vi "Execute.vi"(1 "Numeric":dbl, 4 "Position":i32, 6 "Assembly Type":string, 8 "error in (no error)":errorcluster, 9 "Workspace":T1, 10 "Cluster":T2={"I-O.lvclass"=refnum, "Gantry"=refnum, "Dispenser"="COM1"}, 11 "Pick and Place in":refnum<class "Pick and Place.lvclass">) -> (0 "error out":errorcluster, 2 "Control Out":T2={"I-O.lvclass"=refnum, "Gantry"=refnum, "Dispenser"="COM1"}, 3 "Pick and Place out":refnum<class "Pick and Place.lvclass">)   [LabVIEW 2021, in "Pick and Place.lvclass"]
uses:
  Pick and Place.lvclass
  Controller/Controllers.ctl
  Controller/I-O/I-O.lvclass
  C:/Program Files (x86)/Aerotech/A3200/LabVIEW/2010/Bin/Aerotech.A3200.dll
  Program Files (x86)/Aerotech/A3200/LabVIEW/2010/Bin/Aerotech.A3200.dll
  Workspace/Workspace.ctl
  Pick and Place.lvclass/Pick and Place.ctl
  Pick and Place Type.ctl
  Drivers/Aerotech A3200/Parameters/GetAxisParameterDouble.vi
  Controller/Motion/Motion.lvclass
  Controller/Motion/A3200/A3200.lvclass
  Drivers/Aerotech A3200/Aerotech.lvlib
  Controller/Controller.lvclass
  Workspace/Fixture.lvclass
panel:
  out "Seconary Pickup time 2":timestamp
  out "Seconary Pickup time 1":timestamp
  out "milliseconds to wait":u32
  out "XYZTheta Out":dbl[](array[numeric])
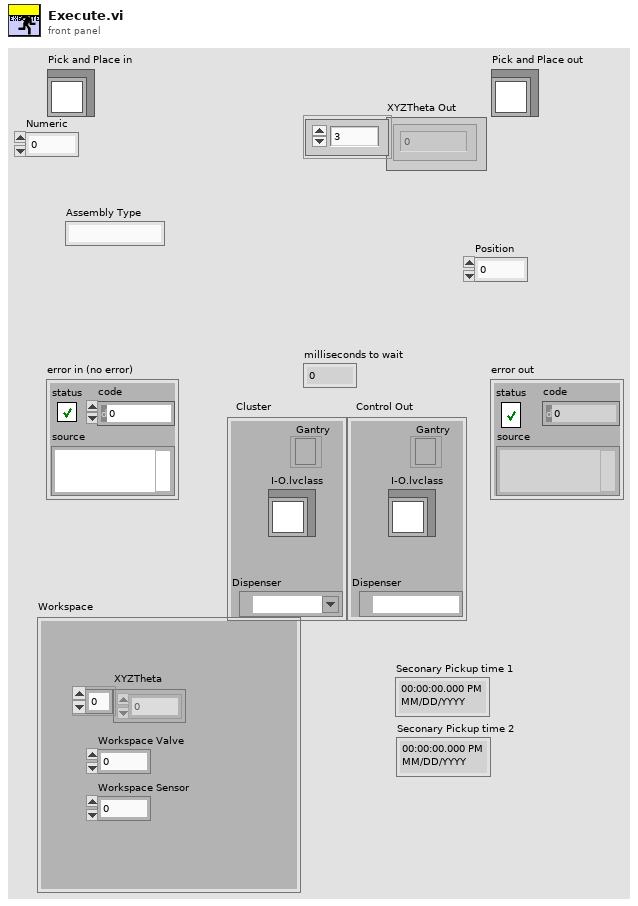
[diagram p1: front panel]
types:
  T1 = typedef "Fixture.lvclass/Workspace.ctl" = cluster{"XYZTheta":dbl[], "Workspace Valve":i32, "Workspace Sensor":i32}
  T2 = typedef "Controller.lvclass/Controllers.ctl" = cluster{"I-O.lvclass":refnum<class "I-O.lvclass">, "Gantry":refnum<k24>, "Dispenser":refnum<visa-resource-name>}
  T3 = typedef "I-O.lvclass/Pin Map.ctl" = cluster{"Region Valves":i32[], "Extra Valves":dbl[][][], "Tool Primary Valve":i32, "Tool Secondary Valve":i32, "Region Sensors":i32[], "Extra Sensors":dbl[][][], "Tool Primary Sensor":dbl, "Tool Secondary Sensor":dbl, "Compression Sensor":dbl, "5V":i32, "Dispenser Sensor":dbl}
  T4 = typedef "Pick and Place.lvclass/Pick and Place Type.ctl" = enum16{"Primary Pick Up", "Secondary Pick Up", "Put Down All", "Pick Up All", "Put Down Secondary"}
  T5 = cluster{"Status":bool, "Error Code":i32, "Source":string}
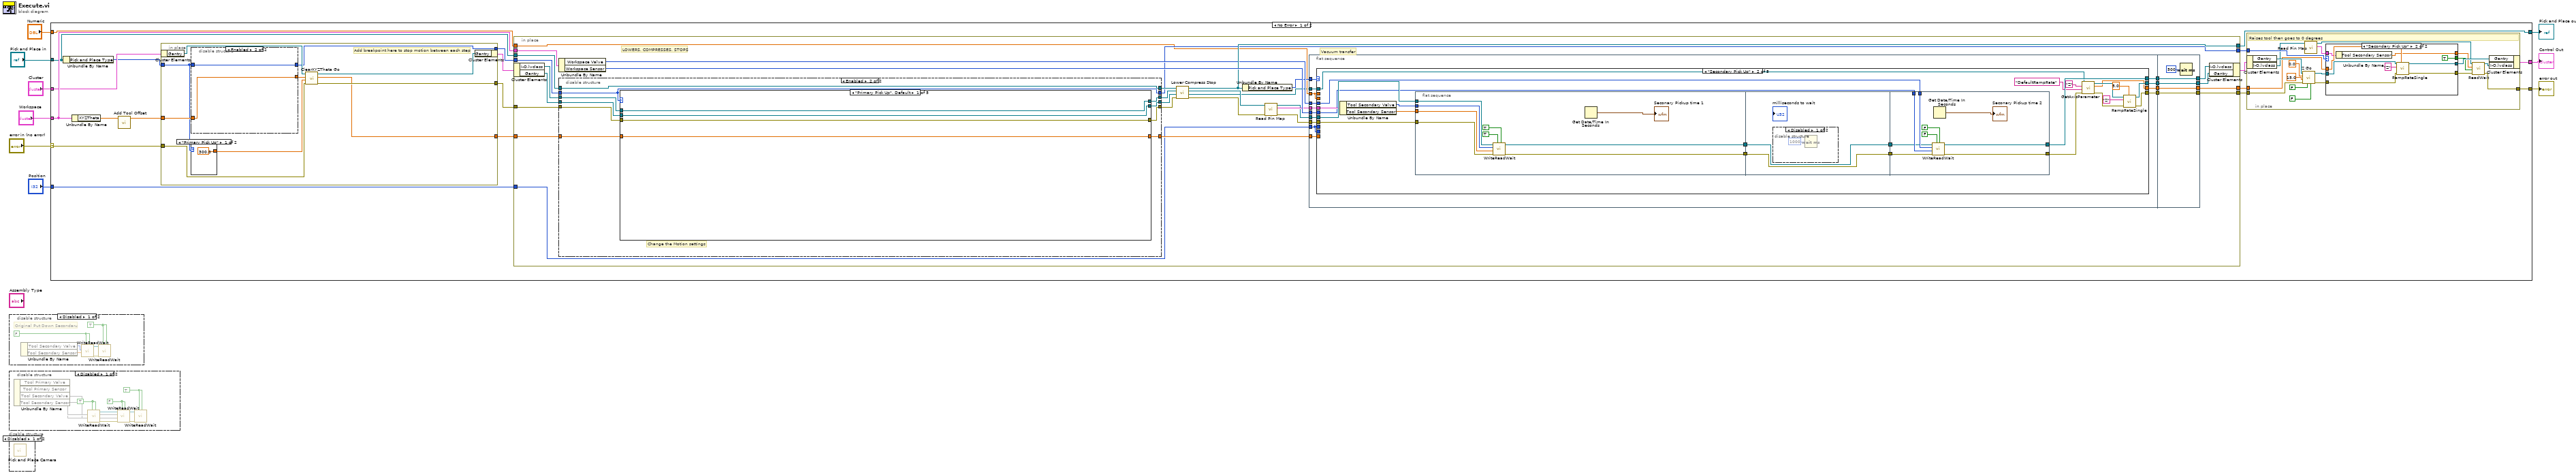
[diagram p0: block diagram]
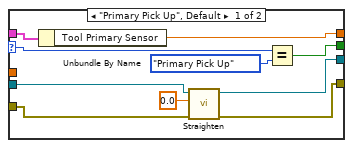
[diagram p5: hidden frame]
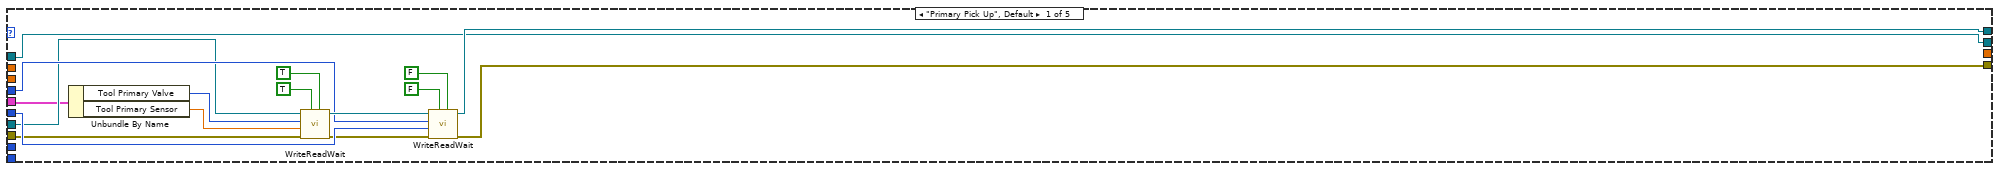
[diagram p6: hidden frame]
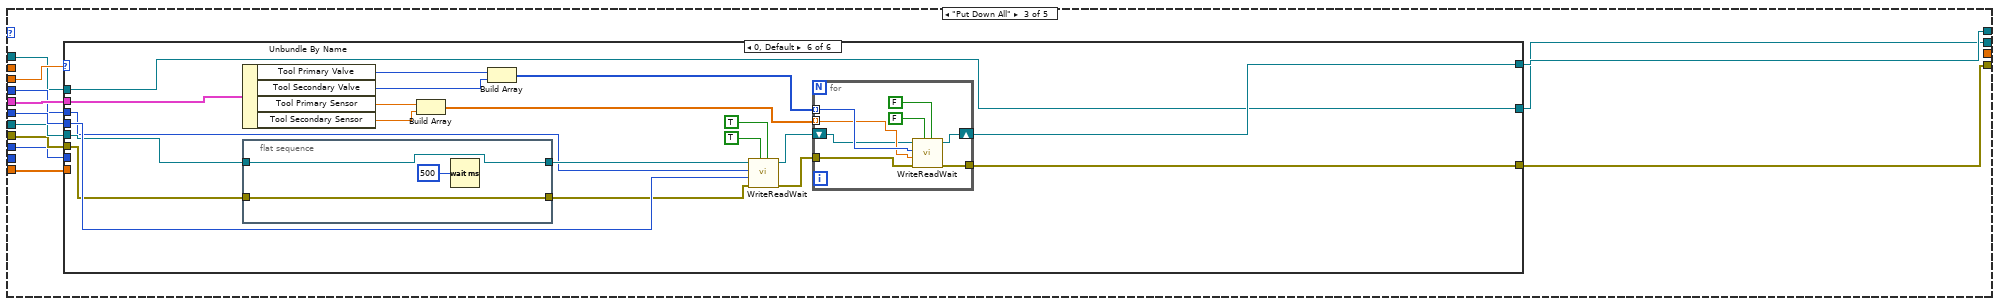
[diagram p8: hidden frame]
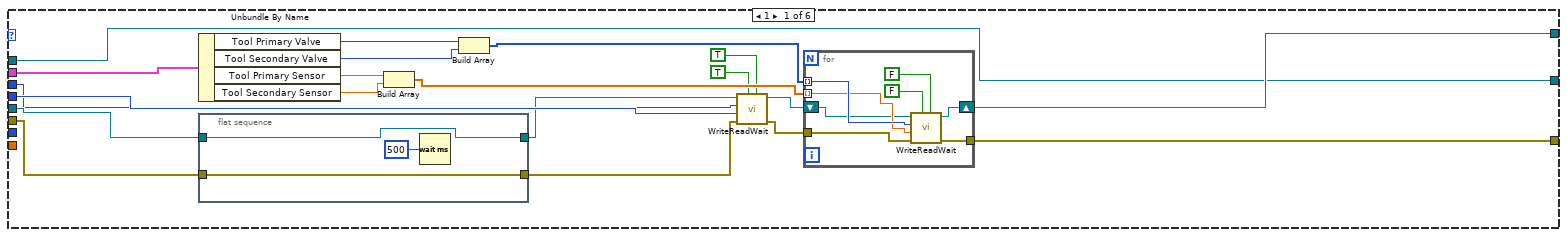
[diagram p9: hidden frame]
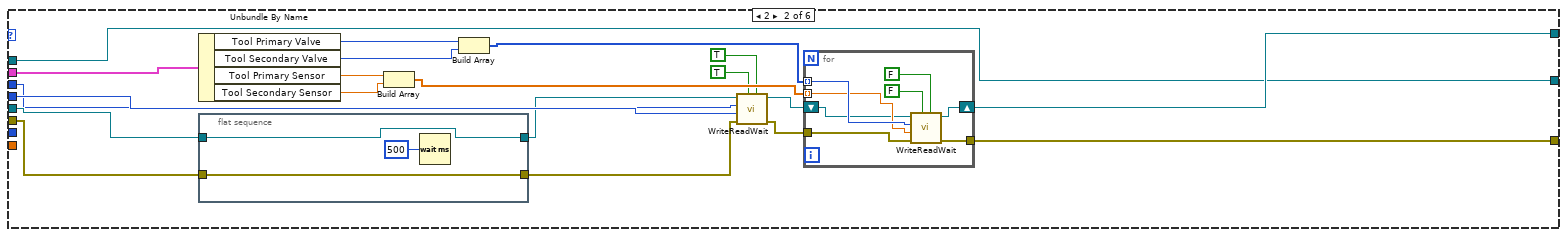
[diagram p10: hidden frame]
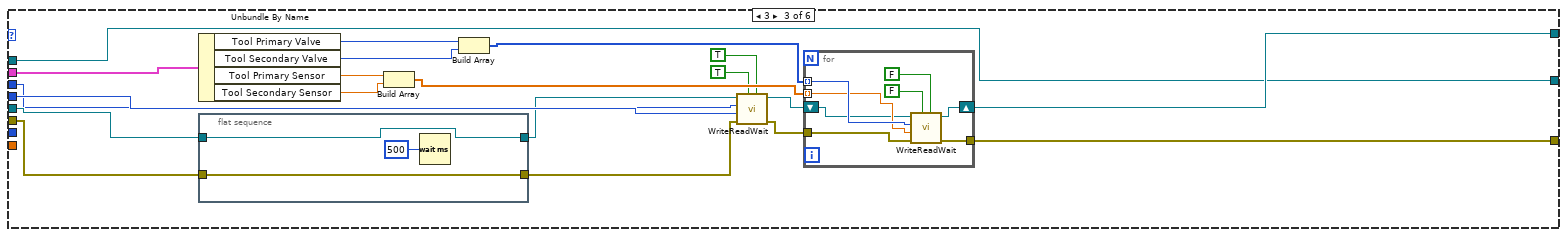
[diagram p11: hidden frame]
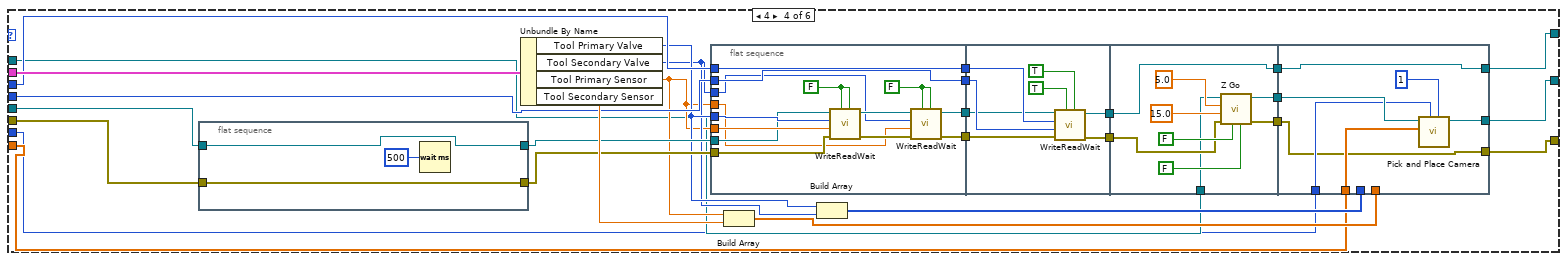
[diagram p12: hidden frame]
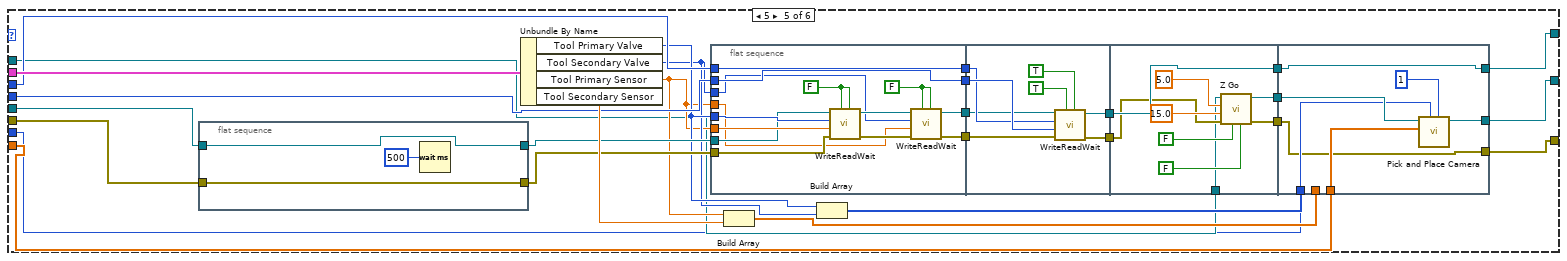
[diagram p13: hidden frame]
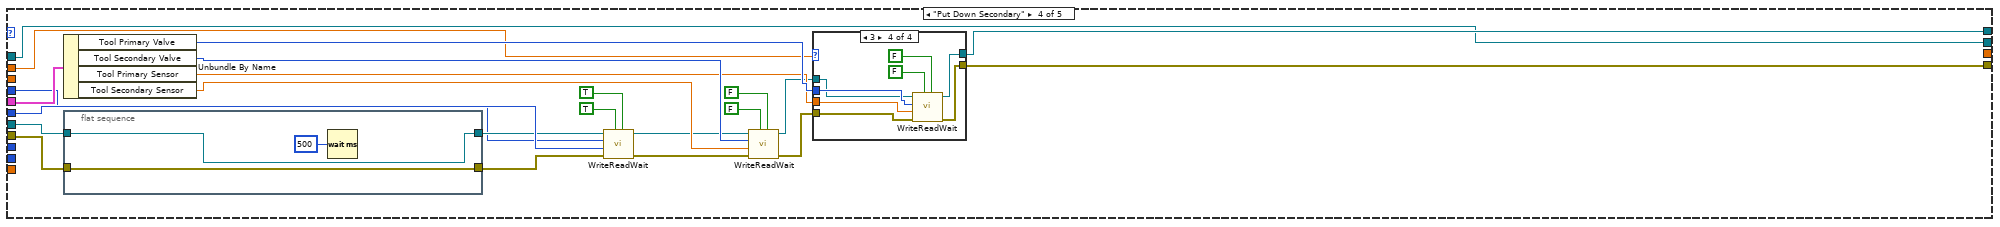
[diagram p14: hidden frame]
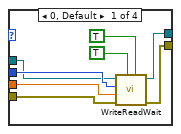
[diagram p15: hidden frame]
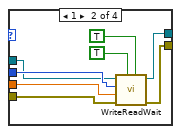
[diagram p16: hidden frame]
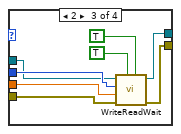
[diagram p17: hidden frame]
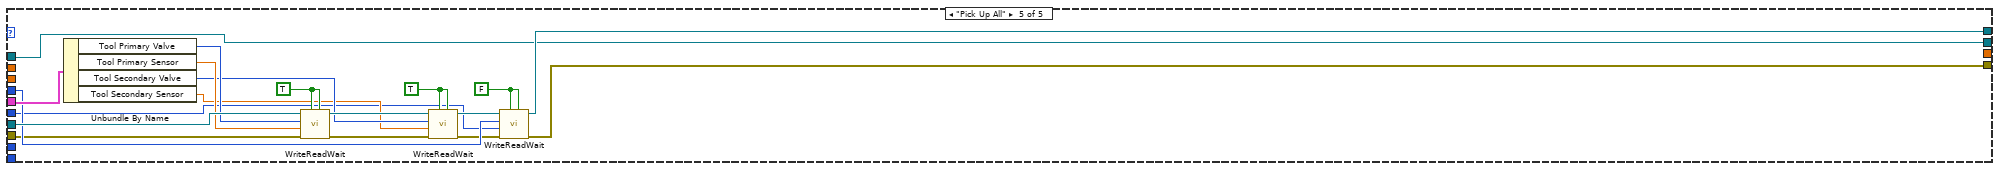
[diagram p18: hidden frame]
diagram:
  n1 = disable-structure shown="Disabled" {
    frame Disabled {
      w14 = TRUE ("Read Value")
      w18 = FALSE ("Write Value")
      # "Original Put Down Secondaru"
      n2 = Unbundle By Name() -> ("Tool Secondary Valve"=w20:i32, "Tool Secondary Sensor"=w19:dbl)  [unwired: 1 in]
      n3 = call "WriteReadWait.vi"("Read Value"=w18, "Write Value"=w18, "Read"=w19, "Write"=w20) -> ("error out"=w11:errorcluster, "I-O out"=w17:refnum<class "I-O.lvclass">, "error in (no error)"=w12:errorcluster, "I-O in"=w21:refnum<class "I-O.lvclass">)  [unwired: 4 in]
      n4 = call "WriteReadWait.vi"("Read Value"=w14, "Write Value"=w14, "error in (no error)"=w11, "I-O in"=w17) -> ("error out"=w10:errorcluster, "I-O out"=w13:refnum<class "I-O.lvclass">, "Read"=w15:i32, "Write"=w16:i32)  [unwired: 4 in]
    }
    frame Enabled {
    }
  }
  n5 = disable-structure shown="Disabled" {
    frame Disabled {
      w27 = TRUE ("Read Value")
      w31 = FALSE ("Write Value")
      w37 = TRUE ("Write Value")
      n6 = Unbundle By Name() -> (w39:T3, "Tool Primary Valve"=w36, "Tool Primary Sensor"=w35, "Tool Secondary Valve"=w33, "Tool Secondary Sensor"=w32)
      n7 = call "WriteReadWait.vi"("Read Value"=w37, "Write Value"=w37, "Read"=w35, "Write"=w36) -> ("error out"=w24:errorcluster, "I-O out"=w34:refnum<class "I-O.lvclass">, "error in (no error)"=w25:errorcluster, "I-O in"=w38:refnum<class "I-O.lvclass">)  [unwired: 4 in]
      n8 = call "WriteReadWait.vi"("Read Value"=w31, "Write Value"=w31, "error in (no error)"=w24, "Read"=w32, "Write"=w33, "I-O in"=w34) -> ("error out"=w23:errorcluster, "I-O out"=w30:refnum<class "I-O.lvclass">)  [unwired: 4 in]
      n9 = call "WriteReadWait.vi"("Read Value"=w27, "Write Value"=w27, "error in (no error)"=w23, "I-O in"=w30) -> ("error out"=w22:errorcluster, "I-O out"=w26:refnum<class "I-O.lvclass">, "Read"=w28:i32, "Write"=w29:i32)  [unwired: 4 in]
    }
    frame Enabled {
    }
  }
  n10 = disable-structure shown="Disabled" {
    frame Disabled {
      n11 = call "Pick and Place Camera.vi"() -> ("Gantry In"=w40:refnum<k24>, "XYZTheta"=w41:dbl[], "Position"=w44:i32, "Tray Number"=w43:i32, "Gantry Out"=w42:refnum<k24>)  [unwired: 6 in]
    }
    frame Enabled {
    }
  }
  n12 = case shown="No Error" "error in (no error)" {
    selector: "error in (no error)" -> [w58 w662]
    tunnel: "Cluster" -> [w62 w663]
    tunnel: "Workspace" -> [w63 _]
    tunnel: [w57 w662] -> w3
    tunnel: [w61 w663] -> w4
    tunnel: "Pick and Place in" -> [w53 w661]
    tunnel: [w60 w661] -> w8
    tunnel: "Numeric" -> [w47 _]
    tunnel: "Position" -> [w46 _]
    frame No Error {
      n13 = Unbundle By Name(w53) -> ("Pick and Place Type"=w52:T4)
      n14 = Unbundle By Name(w63) -> ("XYZTheta"=w49:dbl[])
      n15 = call "Add Tool Offset.vi"("XYZTheta"=w49) -> ("Array"=w59:dbl[])  [unwired: 10 in]
      n16 = in-place "In Place Element Structure" {
        in-place-border: w59 -> [w642]
        in-place-border: w58 -> [w643]
        in-place-border: [w644] -> w55
        in-place-border: w52 -> [w638]
        in-place-border: [w640] -> w51
        in-place-border: [w639] -> w48
        # "Add breakpoint here to stop motion between each step"
        n17 = in-place-cluster #1(w62) -> ("Gantry"=w646:refnum<k24>)
        n18 = disable-structure shown="Enabled" {
          disable-tunnel: w638 -> [w649 w659]
          disable-tunnel: w642 -> [w651 w660]
          disable-tunnel: [w650 w660] -> w641
          disable-tunnel: [w649 w659] -> w640
          frame Disabled {
            n19 = case shown="\"Put Down All\"" w649 {
              tunnel: w651 -> [w652 w655]
              tunnel: [w652 w653] -> w650
              frame "Primary Pick Up", Default {
              }
              frame "Put Down All" {
                n20 = in-place {
                  n21 = in-place-array #2(w655, 3) -> (w658:dbl)
                  n22 = Add(x=w658, y=1.5707963267948966) -> (x+y=w656:dbl)
                  n23 = in-place-array #2(w656) -> (w653:dbl[])  [unwired: 1 out]
                }
              }
            }
          }
          frame Enabled {
          }
        }
        n24 = case shown="\"Primary Pick Up\"" w638 {
          tunnel: [300.0 ("Speed") 100.0 ("Speed")] -> w637
          frame "Primary Pick Up" {
          }
          frame "Secondary Pick Up", Default {
          }
        }
        n25 = call "ClearXYZTheta Go.vi"("error in (no error)"=w643, "Speed"=w637, "XYZTheta In"=w641, "Gantry In"=w646) -> ("error out"=w644:errorcluster, "XYZTheta Out"=w639:dbl[], "Gantry Out"=w645:refnum<k24>)  [unwired: 5 in]
        n26 = in-place-cluster #1("Gantry"=w645) -> (w64:T2)
      }
      n27 = in-place {
        in-place-border: w63 -> [w135]
        in-place-border: w53 -> [w124]
        in-place-border: [w129] -> w60
        in-place-border: w55 -> [w120]
        in-place-border: [w126] -> w54
        in-place-border: w51 -> [w118]
        in-place-border: [w113] -> w50
        in-place-border: w48 -> [w115]
        in-place-border: w47 -> [w112]
        in-place-border: w46 -> [w108]
        in-place-border: [w107] -> w45
        # "Vacuum transfer"
        # "LOWERS, COMPRESSES, STOPS"
        n28 = in-place-cluster #3(w64) -> ("I-O.lvclass"=w123:refnum<class "I-O.lvclass">, "Gantry"=w121:refnum<k24>)
        n29 = Unbundle By Name(w135) -> ("Workspace Valve"=w117:i32, "Workspace Sensor"=w134:i32)
        n30 = disable-structure shown="Enabled" {
          disable-tunnel: [w570 w580] -> w125
          disable-tunnel: w124 -> [w570 w580]
          disable-tunnel: w123 -> [w569 w579]
          disable-tunnel: [w569 w578] -> w122
          disable-tunnel: w121 -> [w568 w574]
          disable-tunnel: w120 -> [w567 w577]
          disable-tunnel: [w567 w576] -> w119
          disable-tunnel: w118 -> [w566 w572]
          disable-tunnel: [_ w575] -> w116
          disable-tunnel: w115 -> [_ w573]
          disable-tunnel: [_ w572] -> w113
          disable-tunnel: [_ w571] -> w111
          frame Disabled {
          }
          frame Enabled {
            # "Change the Motion settings"
            n31 = case shown="\"Primary Pick Up\", Default" w572 {
              tunnel: w579 -> [w584 w588 w592 w596 w636]
              tunnel: [w584 w588 w592 w596 w636] -> w578
              tunnel: w577 -> [w583 w587 w591 w595 w628]
              tunnel: [w583 w587 w591 w595 w605] -> w576
              tunnel: [w582 w586 w590 w594 w604] -> w575
              tunnel: w574 -> [w582 w586 w590 w594 w630]
              tunnel: w573 -> [w581 w585 w589 w593 w635]
              tunnel: [w581 w585 w589 w593 w597] -> w571
              frame "Primary Pick Up", Default {
              }
              frame "Secondary Pick Up" {
              }
              frame "Put Down All" {
              }
              frame "Pick Up All" {
              }
              frame "Put Down Secondary" {
                w631 = dbl[] [0.0, 0.0, 0.0, 0.0] ("y")
                w632 = dbl[] [0.0, 0.0, 0.0, 0.0] ("y")
                w633 = dbl[] [0.0, 0.0, 0.0, 0.0] ("y")
                w634 = dbl[] [0.0, 0.0, 0.0, 0.0] ("y")
                # "at 33 mm normally"
                # "In Radians\n\npositive = Clockwise\nNegative = Counterclockwise\n\n0.174533 = 10 degrees"
                # "Theta Motion"
                # "0 is the left side\nPositive = Go Right\nNegative = Go Left"
                # "0 is the back\nPositive = Go Forward\nNegative = Go Backwards"
                # "0 is top, about 80 is the tray\npositive = Go Down\nNegative = Go Up"
                # "Z Motion"
                # "Y Motion"
                # "X Motion"
                n32 = disable-structure shown="Disabled" {
                  frame Disabled {
                    n33 = call "ClearXYZTheta Go.vi"() -> ()  [unwired: 9 in, 3 out]
                  }
                  frame Enabled {
                  }
                }
                n34 = Add(x=w635, y=w634) -> (x+y=w629:dbl[])
                n35 = call "XYZThetaGo.vi"("error in (no error)"=w628, "XYZTheta In"=w629, "Gantry In"=w630) -> ("error out"=w624:errorcluster, "XYZTheta Out"=w627:dbl[], "Gantry Out"=w626:refnum<k24>)  [unwired: 6 in]
                n36 = Subtract(x=w627, y=w634) -> (x-y=w625:dbl[])
                n37 = call "XYZThetaGo.vi"("error in (no error)"=w624, "XYZTheta In"=w625, "Gantry In"=w626) -> ("error out"=w601:errorcluster, "XYZTheta Out"=w623:dbl[], "Gantry Out"=w603:refnum<k24>)  [unwired: 6 in]
                n38 = Add(x=w623, y=w633) -> (x+y=w602:dbl[])
                n39 = call "XYZThetaGo.vi"("error in (no error)"=w601, "XYZTheta In"=w602, "Gantry In"=w603) -> ("error out"=w600:errorcluster, "XYZTheta Out"=w599:dbl[], "Gantry Out"=w598:refnum<k24>)  [unwired: 6 in]
                n40 = Subtract(x=w599, y=w633) -> (x-y=w621:dbl[])
                n41 = call "XYZThetaGo.vi"("error in (no error)"=w600, "XYZTheta In"=w621, "Gantry In"=w598) -> ("error out"=w617:errorcluster, "XYZTheta Out"=w622:dbl[], "Gantry Out"=w620:refnum<k24>)  [unwired: 6 in]
                n42 = Add(x=w622, y=w632) -> (x+y=w618:dbl[])
                n43 = call "XYZThetaGo.vi"("error in (no error)"=w617, "XYZTheta In"=w618, "Gantry In"=w620) -> ("error out"=w614:errorcluster, "XYZTheta Out"=w619:dbl[], "Gantry Out"=w616:refnum<k24>)  [unwired: 6 in]
                n44 = Subtract(x=w619, y=w632) -> (x-y=w615:dbl[])
                n45 = call "XYZThetaGo.vi"("error in (no error)"=w614, "XYZTheta In"=w615, "Gantry In"=w616) -> ("error out"=w610:errorcluster, "XYZTheta Out"=w613:dbl[], "Gantry Out"=w612:refnum<k24>)  [unwired: 6 in]
                n46 = Add(x=w613, y=w631) -> (x+y=w611:dbl[])
                n47 = call "XYZThetaGo.vi"("error in (no error)"=w610, "XYZTheta In"=w611, "Gantry In"=w612) -> ("error out"=w606:errorcluster, "XYZTheta Out"=w609:dbl[], "Gantry Out"=w608:refnum<k24>)  [unwired: 6 in]
                n48 = Subtract(x=w609, y=w631) -> (x-y=w607:dbl[])
                n49 = call "XYZThetaGo.vi"("error in (no error)"=w606, "XYZTheta In"=w607, "Gantry In"=w608) -> ("error out"=w605:errorcluster, "XYZTheta Out"=w597:dbl[], "Gantry Out"=w604:refnum<k24>)  [unwired: 6 in]
                "XYZTheta Out" <- w597
              }
            }
          }
        }
        n50 = call "Lower Compress Stop.vi"("error in (no error)"=w119, "Gantry In"=w116, "I-O.lvclass"=w122, "Pick and Place in"=w125) -> ("error out"=w128:errorcluster, "Gantry Out"=w110:refnum<k24>, "I-O out"=w130:refnum<class "I-O.lvclass">, "Pick and Place Out"=w129:refnum<class "Pick and Place.lvclass">)  [unwired: 4 in]
        n51 = Unbundle By Name(w129) -> ("Pick and Place Type"=w114:T4)
        n52 = call-dynamic "Read Pin Map.vi"("error in (no error)"=w128, "I-O in"=w130) -> ("error out"=w127:errorcluster, "Pin Map 2"=w133:T3, "I-O out"=w132:refnum<class "I-O.lvclass">)  [unwired: 7 in]
        n53 = flat-sequence {
          tunnel: w134 -> [w149]
          tunnel: w133 -> [w148]
          tunnel: w132 -> [w147]
          tunnel: w127 -> [w145]
          tunnel: w117 -> [w143]
          tunnel: w114 -> [w142]
          tunnel: w112 -> [w141]
          tunnel: w111 -> [w140]
          tunnel: w110 -> [w139]
          tunnel: w108 -> [w137]
          tunnel: [w146] -> w106
          tunnel: [w144] -> w105
          tunnel: [w138] -> w104
          tunnel: [w136] -> w103
          tunnel: [w562] -> w107
          tunnel: [w563] -> w109
          tunnel: [w564] -> w126
          tunnel: [w565] -> w131
          tunnel: w106 -> [w565]
          tunnel: w105 -> [w564]
          tunnel: w104 -> [w563]
          tunnel: w103 -> [w562]
          frame #0 {
            n54 = case shown="\"Secondary Pick Up\"" w142 {
              tunnel: w143 -> [w163 w178 w215 w496 w550]
              tunnel: w149 -> [w162 w179 w220 w503 w549]
              tunnel: [w157 w177 w221 w506 w547] -> w146
              tunnel: w147 -> [w156 w186 w218 w500 w559]
              tunnel: w148 -> [w155 w185 w219 w502 w560]
              tunnel: w145 -> [w153 w184 w217 w498 w546]
              tunnel: [w151 w174 w216 w497 w543] -> w144
              tunnel: w141 -> [_ _ _ w485 _]
              tunnel: w141 -> [_ _ w214 _ _]
              tunnel: w140 -> [_ _ w213 _ _]
              tunnel: w137 -> [_ _ _ _ _]
              tunnel: w139 -> [w150 w170 w212 w484 w542]
              tunnel: [w150 w176 w211 w484 w542] -> w138
              tunnel: w137 -> [_ _ w210 _ _]
              tunnel: [_ w166 _ _ _] -> w136
              frame "Primary Pick Up", Default {
                n55 = Unbundle By Name(w155) -> ("Tool Primary Valve"=w154:i32, "Tool Primary Sensor"=w165:dbl)
                n56 = call "WriteReadWait.vi"("Read Value"=TRUE, "Write Value"=TRUE, "error in (no error)"=w153, "Read"=w165, "Write"=w154, "I-O in"=w156) -> ("error out"=w152:errorcluster, "I-O out"=w164:refnum<class "I-O.lvclass">)  [unwired: 4 in]
                n57 = call "WriteReadWait.vi"("Read Value"=FALSE ("Write Value"), "Write Value"=FALSE ("Read Value"), "error in (no error)"=w152, "Read"=w162, "Write"=w163, "I-O in"=w164) -> ("error out"=w151:errorcluster, "I-O out"=w157:refnum<class "I-O.lvclass">)  [unwired: 4 in]
              }
              frame "Secondary Pick Up" {
                n58 = Unbundle By Name(w185) -> ("Tool Secondary Valve"=w188:i32, "Tool Secondary Sensor"=w187:dbl)
                n59 = flat-sequence {
                  tunnel: w188 -> [w194]
                  tunnel: w187 -> [w193]
                  tunnel: w186 -> [w192]
                  tunnel: w184 -> [w191]
                  tunnel: [w197] -> w183
                  tunnel: [w190] -> w182
                  tunnel: w183 -> [w199]
                  tunnel: w182 -> [w198]
                  tunnel: [w199] -> w181
                  tunnel: [w198] -> w180
                  tunnel: w181 -> [w206]
                  tunnel: w180 -> [w209]
                  tunnel: w179 -> [w208]
                  tunnel: w178 -> [w207]
                  tunnel: [w205] -> w168
                  tunnel: [w204] -> w177
                  frame #0 {
                    n60 = call "WriteReadWait.vi"("Read Value"=TRUE, "Write Value"=TRUE, "error in (no error)"=w191, "Read"=w193, "Write"=w194, "I-O in"=w192) -> ("error out"=w190:errorcluster, "I-O out"=w197:refnum<class "I-O.lvclass">)  [unwired: 4 in]
                    n61 = Get Date/Time In Seconds() -> (seconds since 1Jan1904=→"Seconary Pickup time 1":timestamp)
                  }
                  frame #1 {
                    n62 = disable-structure shown="Disabled" {
                      frame Disabled {
                        n63 = Wait (ms)(milliseconds to wait=u32 1000) -> ()  [unwired: 1 out]
                      }
                      frame Enabled {
                      }
                    }
                  }
                  frame #2 {
                    n64 = call "WriteReadWait.vi"("Read Value"=FALSE ("Write Value"), "Write Value"=FALSE ("Read Value"), "error in (no error)"=w209, "Read"=w208, "Write"=w207, "I-O in"=w206) -> ("error out"=w205:errorcluster, "I-O out"=w204:refnum<class "I-O.lvclass">)  [unwired: 4 in]
                    n65 = Get Date/Time In Seconds() -> (seconds since 1Jan1904=→"Seconary Pickup time 2":timestamp)
                  }
                }
                n66 = call-poly "GetAxisParameter.vi"("error in (no error)"=w168, "Parameter Name"="DefaultRampRate", "axis name"="Z", "controller in"=w170) -> ("error out"=w167:errorcluster, "value"=w166:dbl, "controller out"=w169:refnum<k24>)  [unwired: 5 in]
                n67 = call "RampRateSingle.vi"("ramp rate"=5.0, "error in (no error)"=w167, "axis name"="Z", "controller in"=w169) -> ("error out (no error)"=w174:T5, "controller out"=w176:refnum<k24>)  [unwired: 6 in]
              }
              frame "Put Down All" {
                n68 = case shown="0, Default" w214 {
                  tunnel: [w235 w266 w297 w332 w401 w466] -> w221
                  tunnel: w220 -> [w232 w263 w294 w341 w410 w463]
                  tunnel: w219 -> [w231 w262 w293 w340 w409 w462]
                  tunnel: w218 -> [w228 w259 w290 w338 w407 w459]
                  tunnel: w217 -> [w225 w256 w287 w336 w405 w456]
                  tunnel: [w224 w255 w286 w331 w400 w455] -> w216
                  tunnel: w215 -> [w223 w254 w285 w335 w404 w454]
                  tunnel: w213 -> [_ _ _ w322 w391 _]
                  tunnel: w212 -> [w222 w253 w284 w327 w396 w453]
                  tunnel: [w222 w253 w284 w323 w392 w453] -> w211
                  tunnel: w210 -> [_ _ _ w321 w390 _]
                  frame 1 {
                    n69 = Unbundle By Name(w231) -> ("Tool Primary Valve"=w236:i32, "Tool Secondary Valve"=w237:i32, "Tool Primary Sensor"=w238:dbl, "Tool Secondary Sensor"=w239:dbl)
                    n70 = flat-sequence {
                      tunnel: [w243] -> w229
                      tunnel: w228 -> [w243]
                      tunnel: [w242] -> w226
                      tunnel: w225 -> [w242]
                      frame #0 {
                        # "Delay After Placing"
                        n71 = Wait (ms)(milliseconds to wait=u32 500) -> ()  [unwired: 1 out]
                      }
                    }
                    n72 = Build Array(w238, w239) -> (w241:dbl[])
                    n73 = Build Array(w236, w237) -> (w240:i32[])
                    n74 = call "WriteReadWait.vi"("Read Value"=TRUE, "Write Value"=TRUE, "error in (no error)"=w226, "Read"=w232, "Write"=w223, "I-O in"=w229) -> ("error out"=w227:errorcluster, "I-O out"=w230:refnum<class "I-O.lvclass">)  [unwired: 4 in]
                    n75 = for {
                      shift-right: [w247] -> w235
                      shift-left: w230 -> [w248]
                      tunnel: w240 -> [w250] mode=indexing
                      tunnel: w241 -> [w249] mode=indexing
                      tunnel: w227 -> [w246]
                      tunnel: [w245] -> w224
                      n76 = call "WriteReadWait.vi"("Read Value"=FALSE ("Write Value"), "Write Value"=FALSE ("Read Value"), "error in (no error)"=w246, "Read"=w249, "Write"=w250, "I-O in"=w248) -> ("error out"=w245:errorcluster, "I-O out"=w247:refnum<class "I-O.lvclass">)  [unwired: 4 in]
                    }
                  }
                  frame 2 {
                    n77 = Unbundle By Name(w262) -> ("Tool Primary Valve"=w267:i32, "Tool Secondary Valve"=w268:i32, "Tool Primary Sensor"=w269:dbl, "Tool Secondary Sensor"=w270:dbl)
                    n78 = flat-sequence {
                      tunnel: [w274] -> w260
                      tunnel: w259 -> [w274]
                      tunnel: [w273] -> w257
                      tunnel: w256 -> [w273]
                      frame #0 {
                        # "Delay After Placing"
                        n79 = Wait (ms)(milliseconds to wait=u32 500) -> ()  [unwired: 1 out]
                      }
                    }
                    n80 = Build Array(w269, w270) -> (w272:dbl[])
                    n81 = Build Array(w267, w268) -> (w271:i32[])
                    n82 = call "WriteReadWait.vi"("Read Value"=TRUE, "Write Value"=TRUE, "error in (no error)"=w257, "Read"=w263, "Write"=w254, "I-O in"=w260) -> ("error out"=w258:errorcluster, "I-O out"=w261:refnum<class "I-O.lvclass">)  [unwired: 4 in]
                    n83 = for {
                      shift-right: [w278] -> w266
                      shift-left: w261 -> [w279]
                      tunnel: w271 -> [w281] mode=indexing
                      tunnel: w272 -> [w280] mode=indexing
                      tunnel: w258 -> [w277]
                      tunnel: [w276] -> w255
                      n84 = call "WriteReadWait.vi"("Read Value"=FALSE ("Write Value"), "Write Value"=FALSE ("Read Value"), "error in (no error)"=w277, "Read"=w280, "Write"=w281, "I-O in"=w279) -> ("error out"=w276:errorcluster, "I-O out"=w278:refnum<class "I-O.lvclass">)  [unwired: 4 in]
                    }
                  }
                  frame 3 {
                    n85 = Unbundle By Name(w293) -> ("Tool Primary Valve"=w298:i32, "Tool Secondary Valve"=w299:i32, "Tool Primary Sensor"=w300:dbl, "Tool Secondary Sensor"=w301:dbl)
                    n86 = flat-sequence {
                      tunnel: [w305] -> w291
                      tunnel: w290 -> [w305]
                      tunnel: [w304] -> w288
                      tunnel: w287 -> [w304]
                      frame #0 {
                        # "Delay After Placing"
                        n87 = Wait (ms)(milliseconds to wait=u32 500) -> ()  [unwired: 1 out]
                      }
                    }
                    n88 = Build Array(w300, w301) -> (w303:dbl[])
                    n89 = Build Array(w298, w299) -> (w302:i32[])
                    n90 = call "WriteReadWait.vi"("Read Value"=TRUE, "Write Value"=TRUE, "error in (no error)"=w288, "Read"=w294, "Write"=w285, "I-O in"=w291) -> ("error out"=w289:errorcluster, "I-O out"=w292:refnum<class "I-O.lvclass">)  [unwired: 4 in]
                    n91 = for {
                      shift-right: [w309] -> w297
                      shift-left: w292 -> [w310]
                      tunnel: w302 -> [w312] mode=indexing
                      tunnel: w303 -> [w311] mode=indexing
                      tunnel: w289 -> [w308]
                      tunnel: [w307] -> w286
                      n92 = call "WriteReadWait.vi"("Read Value"=FALSE ("Write Value"), "Write Value"=FALSE ("Read Value"), "error in (no error)"=w308, "Read"=w311, "Write"=w312, "I-O in"=w310) -> ("error out"=w307:errorcluster, "I-O out"=w309:refnum<class "I-O.lvclass">)  [unwired: 4 in]
                    }
                  }
                  frame 4 {
                    n93 = flat-sequence {
                      tunnel: [w382] -> w339
                      tunnel: w338 -> [w382]
                      tunnel: [w381] -> w337
                      tunnel: w336 -> [w381]
                      frame #0 {
                        # "Delay After Placing"
                        n94 = Wait (ms)(milliseconds to wait=u32 500) -> ()  [unwired: 1 out]
                      }
                    }
                    n95 = Unbundle By Name(w340) -> ("Tool Primary Valve"=w330:i32, "Tool Secondary Valve"=w329:i32, "Tool Primary Sensor"=w328:dbl, "Tool Secondary Sensor"=w342:dbl)
                    n96 = flat-sequence {
                      tunnel: w335 -> [w355]
                      tunnel: w337 -> [w349]
                      tunnel: w339 -> [w352]
                      tunnel: w341 -> [w356]
                      tunnel: [w356] -> w320
                      tunnel: [w350] -> w319
                      tunnel: [w347] -> w317
                      tunnel: [w355] -> w315
                      tunnel: w330 -> [w354]
                      tunnel: w328 -> [w353]
                      tunnel: w329 -> [w346]
                      tunnel: w328 -> [w345]
                      tunnel: w320 -> [w364]
                      tunnel: w319 -> [w362]
                      tunnel: [w361] -> w318
                      tunnel: w317 -> [w358]
                      tunnel: [w357] -> w316
                      tunnel: w315 -> [w363]
                      tunnel: w318 -> [w373]
                      tunnel: [w373] -> w326
                      tunnel: w316 -> [w368]
                      tunnel: [w367] -> w325
                      tunnel: w327 -> [w366]
                      tunnel: [w365] -> w324
                      tunnel: w334 -> [_]
                      tunnel: w333 -> [_]
                      tunnel: [w374] -> w332
                      tunnel: [w375] -> w331
                      tunnel: w321 -> [w377]
                      tunnel: w322 -> [w378]
                      tunnel: [w379] -> w323
                      tunnel: w324 -> [w380]
                      tunnel: w325 -> [w375]
                      tunnel: w326 -> [w374]
                      frame #0 {
                        w344 = FALSE ("Read Value")
                        w343 = FALSE ("Read Value")
                        n97 = call "WriteReadWait.vi"("Read Value"=w344, "Write Value"=w344, "error in (no error)"=w349, "Read"=w353, "Write"=w354, "I-O in"=w352) -> ("error out"=w348:errorcluster, "I-O out"=w351:refnum<class "I-O.lvclass">)  [unwired: 4 in]
                        n98 = call "WriteReadWait.vi"("Read Value"=w343, "Write Value"=w343, "error in (no error)"=w348, "Read"=w345, "Write"=w346, "I-O in"=w351) -> ("error out"=w347:errorcluster, "I-O out"=w350:refnum<class "I-O.lvclass">)  [unwired: 4 in]
                      }
                      frame #1 {
                        n99 = call "WriteReadWait.vi"("Read Value"=TRUE, "Write Value"=TRUE ("Read Value"), "error in (no error)"=w358, "Read"=w364, "Write"=w363, "I-O in"=w362) -> ("error out"=w357:errorcluster, "I-O out"=w361:refnum<class "I-O.lvclass">)  [unwired: 4 in]
                      }
                      frame #2 {
                        n100 = call "Z Go.vi"("Increment"=FALSE, "Return Immediately"=FALSE ("Increment"), "error in (no error)"=w368, "Speed In"=15.0 ("speed"), "Position In"=5.0 ("position"), "Gantry In"=w366) -> ("error out"=w367:errorcluster, "Gantry Out"=w365:refnum<k24>)  [unwired: 2 in, 2 out]
                      }
                      frame #3 {
                        n101 = call "Pick and Place Camera.vi"("Gantry In"=w380, "XYZTheta"=w378, "Position"=w377, "Tray Number"=1) -> ("Gantry Out"=w379:refnum<k24>)  [unwired: 6 in]
                      }
                    }
                    n102 = Build Array(w328, w342) -> (w333:dbl[])
                    n103 = Build Array(w330, w329) -> (w334:i32[])
                  }
                  frame 5 {
                    n104 = flat-sequence {
                      tunnel: [w451] -> w408
                      tunnel: w407 -> [w451]
                      tunnel: [w450] -> w406
                      tunnel: w405 -> [w450]
                      frame #0 {
                        # "Delay After Placing"
                        n105 = Wait (ms)(milliseconds to wait=u32 500) -> ()  [unwired: 1 out]
                      }
                    }
                    n106 = Unbundle By Name(w409) -> ("Tool Primary Valve"=w399:i32, "Tool Secondary Valve"=w398:i32, "Tool Primary Sensor"=w397:dbl, "Tool Secondary Sensor"=w411:dbl)
                    n107 = flat-sequence {
                      tunnel: w404 -> [w424]
                      tunnel: w406 -> [w418]
                      tunnel: w408 -> [w421]
                      tunnel: w410 -> [w425]
                      tunnel: [w425] -> w389
                      tunnel: [w419] -> w388
                      tunnel: [w416] -> w386
                      tunnel: [w424] -> w384
                      tunnel: w399 -> [w423]
                      tunnel: w397 -> [w422]
                      tunnel: w398 -> [w415]
                      tunnel: w397 -> [w414]
                      tunnel: w389 -> [w433]
                      tunnel: w388 -> [w431]
                      tunnel: [w430] -> w387
                      tunnel: w386 -> [w427]
                      tunnel: [w426] -> w385
                      tunnel: w384 -> [w432]
                      tunnel: w387 -> [w442]
                      tunnel: [w442] -> w395
                      tunnel: w385 -> [w437]
                      tunnel: [w436] -> w394
                      tunnel: w396 -> [w435]
                      tunnel: [w434] -> w393
                      tunnel: w403 -> [_]
                      tunnel: w402 -> [_]
                      tunnel: [w443] -> w401
                      tunnel: [w444] -> w400
                      tunnel: w390 -> [w446]
                      tunnel: w391 -> [w447]
                      tunnel: [w448] -> w392
                      tunnel: w393 -> [w449]
                      tunnel: w394 -> [w444]
                      tunnel: w395 -> [w443]
                      frame #0 {
                        w413 = FALSE ("Read Value")
                        w412 = FALSE ("Read Value")
                        n108 = call "WriteReadWait.vi"("Read Value"=w413, "Write Value"=w413, "error in (no error)"=w418, "Read"=w422, "Write"=w423, "I-O in"=w421) -> ("error out"=w417:errorcluster, "I-O out"=w420:refnum<class "I-O.lvclass">)  [unwired: 4 in]
                        n109 = call "WriteReadWait.vi"("Read Value"=w412, "Write Value"=w412, "error in (no error)"=w417, "Read"=w414, "Write"=w415, "I-O in"=w420) -> ("error out"=w416:errorcluster, "I-O out"=w419:refnum<class "I-O.lvclass">)  [unwired: 4 in]
                      }
                      frame #1 {
                        n110 = call "WriteReadWait.vi"("Read Value"=TRUE, "Write Value"=TRUE ("Read Value"), "error in (no error)"=w427, "Read"=w433, "Write"=w432, "I-O in"=w431) -> ("error out"=w426:errorcluster, "I-O out"=w430:refnum<class "I-O.lvclass">)  [unwired: 4 in]
                      }
                      frame #2 {
                        n111 = call "Z Go.vi"("Increment"=FALSE, "Return Immediately"=FALSE ("Increment"), "error in (no error)"=w437, "Speed In"=15.0 ("speed"), "Position In"=5.0 ("position"), "Gantry In"=w435) -> ("error out"=w436:errorcluster, "Gantry Out"=w434:refnum<k24>)  [unwired: 2 in, 2 out]
                      }
                      frame #3 {
                        n112 = call "Pick and Place Camera.vi"("Gantry In"=w449, "XYZTheta"=w447, "Position"=w446, "Tray Number"=1) -> ("Gantry Out"=w448:refnum<k24>)  [unwired: 6 in]
                      }
                    }
                    n113 = Build Array(w397, w411) -> (w402:dbl[])
                    n114 = Build Array(w399, w398) -> (w403:i32[])
                  }
                  frame 0, Default {
                    n115 = Unbundle By Name(w462) -> ("Tool Primary Valve"=w467:i32, "Tool Secondary Valve"=w468:i32, "Tool Primary Sensor"=w469:dbl, "Tool Secondary Sensor"=w470:dbl)
                    n116 = flat-sequence {
                      tunnel: [w474] -> w460
                      tunnel: w459 -> [w474]
                      tunnel: [w473] -> w457
                      tunnel: w456 -> [w473]
                      frame #0 {
                        # "Delay After Placing"
                        n117 = Wait (ms)(milliseconds to wait=u32 500) -> ()  [unwired: 1 out]
                      }
                    }
                    n118 = Build Array(w469, w470) -> (w472:dbl[])
                    n119 = Build Array(w467, w468) -> (w471:i32[])
                    n120 = call "WriteReadWait.vi"("Read Value"=TRUE, "Write Value"=TRUE, "error in (no error)"=w457, "Read"=w463, "Write"=w454, "I-O in"=w460) -> ("error out"=w458:errorcluster, "I-O out"=w461:refnum<class "I-O.lvclass">)  [unwired: 4 in]
                    n121 = for {
                      shift-right: [w478] -> w466
                      shift-left: w461 -> [w479]
                      tunnel: w471 -> [w481] mode=indexing
                      tunnel: w472 -> [w480] mode=indexing
                      tunnel: w458 -> [w477]
                      tunnel: [w476] -> w455
                      n122 = call "WriteReadWait.vi"("Read Value"=FALSE ("Write Value"), "Write Value"=FALSE ("Read Value"), "error in (no error)"=w477, "Read"=w480, "Write"=w481, "I-O in"=w479) -> ("error out"=w476:errorcluster, "I-O out"=w478:refnum<class "I-O.lvclass">)  [unwired: 4 in]
                    }
                  }
                }
              }
              frame "Put Down Secondary" {
                n123 = Unbundle By Name(w502) -> ("Tool Primary Valve"=w494:i32, "Tool Secondary Valve"=w495:i32, "Tool Primary Sensor"=w492:dbl, "Tool Secondary Sensor"=w493:dbl)
                n124 = flat-sequence {
                  tunnel: [w540] -> w501
                  tunnel: w500 -> [w540]
                  tunnel: [w539] -> w499
                  tunnel: w498 -> [w539]
                  frame #0 {
                    # "Delay After Placing"
                    n125 = Wait (ms)(milliseconds to wait=u32 500) -> ()  [unwired: 1 out]
                  }
                }
                n126 = call "WriteReadWait.vi"("Read Value"=TRUE, "Write Value"=TRUE, "error in (no error)"=w499, "Read"=w503, "Write"=w496, "I-O in"=w501) -> ("error out"=w486:errorcluster, "I-O out"=w487:refnum<class "I-O.lvclass">)  [unwired: 4 in]
                n127 = call "WriteReadWait.vi"("Read Value"=FALSE, "Write Value"=FALSE ("Read Value"), "error in (no error)"=w486, "Read"=w493, "Write"=w495, "I-O in"=w487) -> ("error out"=w488:errorcluster, "I-O out"=w489:refnum<class "I-O.lvclass">)  [unwired: 4 in]
                n128 = case shown="3" w485 {
                  tunnel: [w514 w522 w530 w538] -> w506
                  tunnel: [w513 w521 w529 w537] -> w497
                  tunnel: w494 -> [w512 w520 w528 w536]
                  tunnel: w492 -> [w511 w519 w527 w535]
                  tunnel: w489 -> [w510 w518 w526 w534]
                  tunnel: w488 -> [w507 w515 w523 w531]
                  frame 0, Default {
                    n129 = call "WriteReadWait.vi"("Read Value"=TRUE, "Write Value"=TRUE ("Read Value"), "error in (no error)"=w507, "Read"=w511, "Write"=w512, "I-O in"=w510) -> ("error out"=w513:errorcluster, "I-O out"=w514:refnum<class "I-O.lvclass">)  [unwired: 4 in]
                  }
                  frame 1 {
                    n130 = call "WriteReadWait.vi"("Read Value"=TRUE, "Write Value"=TRUE ("Read Value"), "error in (no error)"=w515, "Read"=w519, "Write"=w520, "I-O in"=w518) -> ("error out"=w521:errorcluster, "I-O out"=w522:refnum<class "I-O.lvclass">)  [unwired: 4 in]
                  }
                  frame 2 {
                    n131 = call "WriteReadWait.vi"("Read Value"=TRUE, "Write Value"=TRUE ("Read Value"), "error in (no error)"=w523, "Read"=w527, "Write"=w528, "I-O in"=w526) -> ("error out"=w529:errorcluster, "I-O out"=w530:refnum<class "I-O.lvclass">)  [unwired: 4 in]
                  }
                  frame 3 {
                    n132 = call "WriteReadWait.vi"("Read Value"=FALSE, "Write Value"=FALSE ("Read Value"), "error in (no error)"=w531, "Read"=w535, "Write"=w536, "I-O in"=w534) -> ("error out"=w537:errorcluster, "I-O out"=w538:refnum<class "I-O.lvclass">)  [unwired: 4 in]
                  }
                }
              }
              frame "Pick Up All" {
                w548 = FALSE ("Read Value")
                w552 = TRUE ("Write Value")
                w558 = TRUE ("Write Value")
                n133 = Unbundle By Name(w560) -> ("Tool Primary Valve"=w557:i32, "Tool Primary Sensor"=w556:dbl, "Tool Secondary Valve"=w554:i32, "Tool Secondary Sensor"=w553:dbl)
                n134 = call "WriteReadWait.vi"("Read Value"=w558, "Write Value"=w558, "error in (no error)"=w546, "Read"=w556, "Write"=w557, "I-O in"=w559) -> ("error out"=w545:errorcluster, "I-O out"=w555:refnum<class "I-O.lvclass">)  [unwired: 4 in]
                n135 = call "WriteReadWait.vi"("Read Value"=w552, "Write Value"=w552, "error in (no error)"=w545, "Read"=w553, "Write"=w554, "I-O in"=w555) -> ("error out"=w544:errorcluster, "I-O out"=w551:refnum<class "I-O.lvclass">)  [unwired: 4 in]
                n136 = call "WriteReadWait.vi"("Read Value"=w548, "Write Value"=w548, "error in (no error)"=w544, "Read"=w549, "Write"=w550, "I-O in"=w551) -> ("error out"=w543:errorcluster, "I-O out"=w547:refnum<class "I-O.lvclass">)  [unwired: 4 in]
              }
            }
          }
          frame #1 {
            n137 = Wait (ms)(milliseconds to wait=500) -> ()  [unwired: 1 out]
          }
        }
        n138 = in-place-cluster #3("I-O.lvclass"=w131, "Gantry"=w109) -> (w56:T2)
      }
      n139 = in-place {
        in-place-border: [w69] -> w57
        in-place-border: w54 -> [w81]
        in-place-border: w50 -> [w74]
        in-place-border: w45 -> [w73]
        # "Raises tool then goes to 0 degrees"
        n140 = in-place-cluster #4(w56) -> ("Gantry"=w78:refnum<k24>, "I-O.lvclass"=w66:refnum<class "I-O.lvclass">)
        n141 = call "Z Go.vi"("Increment"=FALSE, "Return Immediately"=FALSE ("Increment"), "error in (no error)"=w81, "Speed In"=15.0 ("speed"), "Position In"=0.0 ("position"), "Gantry In"=w78) -> ("error out"=w76:errorcluster, "Gantry Out"=w80:refnum<k24>)  [unwired: 2 in, 2 out]
        n142 = call-dynamic "Read Pin Map.vi"("I-O in"=w66) -> ("Pin Map 2"=w67:T3, "I-O out"=w65:refnum<class "I-O.lvclass">)  [unwired: 8 in, 1 out]
        n143 = case shown="\"Secondary Pick Up\"" w74 {
          selector: w74 -> [w89 _]
          tunnel: w80 -> [w93 w101]
          tunnel: [w92 w100] -> w79
          tunnel: w76 -> [w91 w99]
          tunnel: w73 -> [_ w98]
          tunnel: [w87 w97] -> w72
          tunnel: [w86 TRUE] -> w71
          tunnel: [w85 w94] -> w70
          tunnel: w67 -> [w84 w95]
          frame "Primary Pick Up", Default {
            n144 = Unbundle By Name(w84) -> ("Tool Primary Sensor"=w85:dbl)
            n145 = call "Straighten.vi"("error in (no error)"=w91, "Angle (rad)"=0.0, "Gantry In"=w93) -> ("error out"=w87:errorcluster, "Gantry Out"=w92:refnum<k24>)  [unwired: 7 in]
            n146 = Equal?(x=w89, y=Pick_and_Place_Type."Primary Pick Up") -> (x = y?=w86:bool)
          }
          frame "Secondary Pick Up" {
            n147 = Unbundle By Name(w95) -> ("Tool Secondary Sensor"=w94:dbl)
            n148 = call "RampRateSingle.vi"("ramp rate"=w98, "error in (no error)"=w99, "axis name"="Z", "controller in"=w101) -> ("error out (no error)"=w97:T5, "controller out"=w100:refnum<k24>)  [unwired: 6 in]
          }
        }
        n149 = call "ReadWait.vi"("error in (no error)"=w72, "Value"=w71, "Read"=w70, "I-O in"=w65) -> ("error out"=w69:errorcluster, "I-O out"=w68:refnum<class "I-O.lvclass">)  [unwired: 6 in]
        n150 = in-place-cluster #4("Gantry"=w79, "I-O.lvclass"=w68) -> (w61:T2)
      }
    }
    frame Error {
    }
  }
  "error out" <- w3
  "Pick and Place out" <- w8
  "Control Out" <- w4
